vi "Запись в таблицу (SubVI).vi"(1 "data num":u32, 5 "error in":errorcluster, 6 "String Arr in":string[][](array[string]), 7 "Z axis data":dbl, 8 "Шаг измерений":u64, 9 "Y axis data":dbl, 11 "X axis data":dbl) -> (10 "String Arr out":string[][](array[string]), 14 "X axis data out":dbl, 15 "Y axis data out":dbl, 16 "Z axis data out":dbl, 19 "error out":errorcluster)   [LabVIEW 2013]
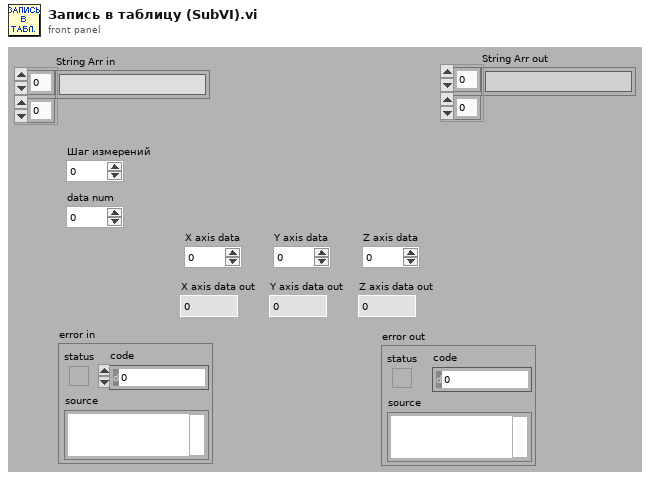
[diagram p1: front panel]
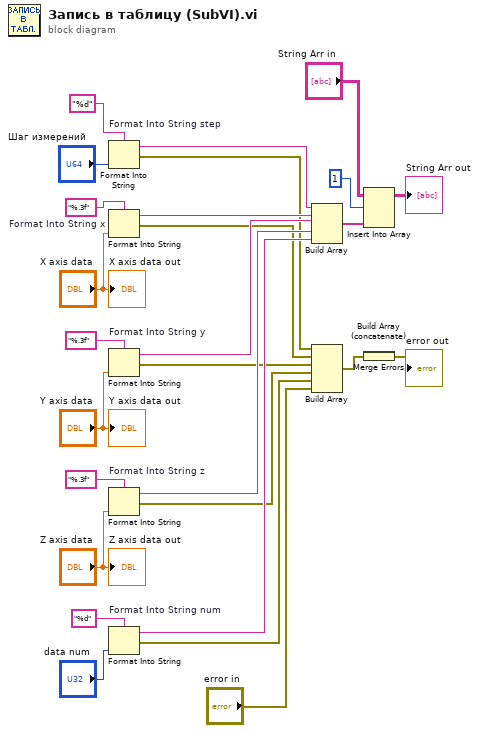
[diagram p0: block diagram]
diagram:
  n1 = Format Into String "Format Into String step"(format string="%d", "Шаг измерений") -> (resulting string=w14:string, error out=w8:errorcluster)  [unwired: 2 in]
  n2 = Format Into String "Format Into String x"(format string="%.3f", "X axis data") -> (resulting string=w13:string, error out=w7:errorcluster)  [unwired: 2 in]
  n3 = Format Into String "Format Into String y"(format string="%.3f", "Y axis data") -> (resulting string=w12:string, error out=w6:errorcluster)  [unwired: 2 in]
  n4 = Format Into String "Format Into String z"(format string="%.3f", "Z axis data") -> (resulting string=w11:string, error out=w5:errorcluster)  [unwired: 2 in]
  n5 = Format Into String "Format Into String num"(format string="%d", "data num") -> (resulting string=w10:string, error out=w4:errorcluster)  [unwired: 2 in]
  n6 = Build Array(w14, w13, w12, w11, w10) -> (w9:string[])
  n7 = Build Array(w8, w7, w6, w5, w4, "error in") -> (w2:errorcluster[])
  n8 = Insert Into Array(array="String Arr in", index (row)=1 ("disabled index (col)"), new element=w9) -> (→"String Arr out":string[][])  [unwired: 1 in]
  n9 = Build Array (concatenate)(w2) -> (w1:errorcluster[])
  n10 = Merge Errors(w1) -> (→"error out":errorcluster)
  "X axis data out" <- "X axis data"
  "Y axis data out" <- "Y axis data"
  "Z axis data out" <- "Z axis data"
